vi "set_origin.vi"(8 "error in (no error)":errorcluster, 11 "StageDL090409Scaffold in":refnum<class "StageDL090409Scaffold.lvclass">) -> (0 "error out":errorcluster, 3 "StageDL090409Scaffold out":refnum<class "StageDL090409Scaffold.lvclass">)   [LabVIEW 2010, in "StageDL090409Scaffold.lvclass"]
uses:
  StageDL090409Scaffold.lvclass
  StageDL090409Scaffold.lvclass/StageDL090409Scaffold.ctl
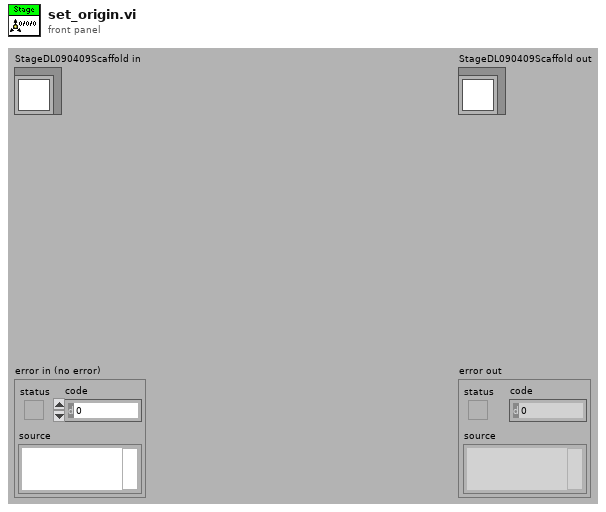
[diagram p1: front panel]
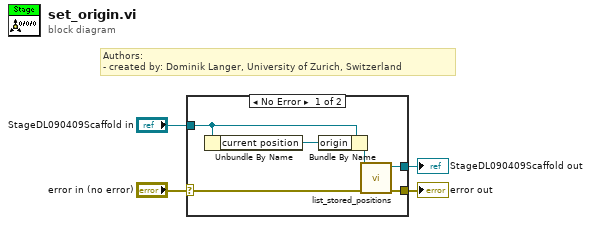
[diagram p0: block diagram]
diagram:
  # "Authors: \n- created by: Dominik Langer, University of Zurich, Switzerland"
  n1 = case shown="No Error" "error in (no error)" {
    selector: "error in (no error)" -> [w8 w12]
    tunnel: [w7 w12] -> w3
    tunnel: [w5 w11] -> w1
    tunnel: "StageDL090409Scaffold in" -> [w10 w11]
    frame No Error {
      n2 = Unbundle By Name(w10) -> ("current position"=w9:refnum<class "SpaceVector.lvclass">)
      n3 = Bundle By Name(cluster=w10, "origin"=w9) -> (w6:refnum<class "StageDL090409Scaffold.lvclass">)
      n4 = call-dynamic "list_stored_positions.vi"("error in (no error)"=w8, "StageDL090409Scaffold in"=w6) -> ("error out"=w7:errorcluster, "StageDL090409Scaffold out"=w5:refnum<class "StageDL090409Scaffold.lvclass">)  [unwired: 8 in]
    }
    frame Error {
    }
  }
  "error out" <- w3
  "StageDL090409Scaffold out" <- w1
